vi "ParseAllClasses.vi"(8 "error in (no error)":errorcluster, 10 "baseClass":refnum<class "baseClass.lvclass">, 11 "CS in":refnum<class "CS.lvclass">) -> (0 "error out":errorcluster, 2 "AllClasses":refnum<class "baseClass.lvclass">[](array[class]), 3 "CS out":refnum<class "CS.lvclass">)   [LabVIEW 2013, in "CS.lvclass"]
uses:
  CS.lvclass
  baseClass/baseClass.lvclass
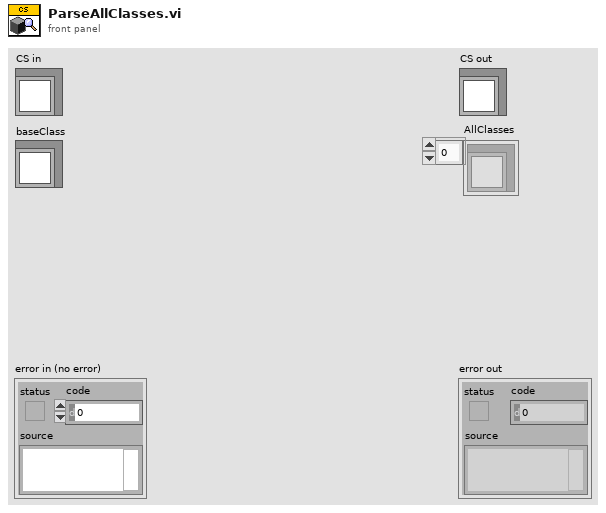
[diagram p1: front panel]
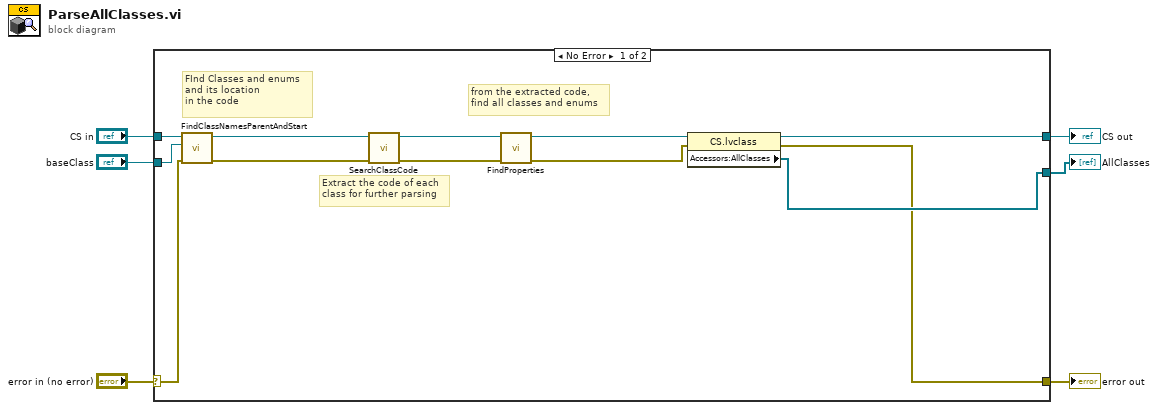
[diagram p0: block diagram]
diagram:
  n1 = case shown="No Error" "error in (no error)" {
    selector: "error in (no error)" -> [w12 w20]
    tunnel: [w11 w20] -> w6
    tunnel: [w15 _] -> w5
    tunnel: [w16 w19] -> w4
    tunnel: "baseClass" -> [w17 _]
    tunnel: "CS in" -> [w18 w19]
    frame No Error {
      # "from the extracted code,\nfind all classes and enums"
      # "Extract the code of each\nclass for further parsing"
      # "FInd Classes and enums\nand its location \nin the code"
      n2 = call "FindClassNamesParentAndStart.vi"("error in (no error)"=w12, "baseClass"=w17, "CS in"=w18) -> ("error out"=w13:errorcluster, "CS out"=w14:refnum<class "CS.lvclass">)  [unwired: 7 in]
      n3 = call-dynamic "SearchClassCode.vi"("error in (no error)"=w13, "CS in"=w14) -> ("error out"=w7:errorcluster, "CS out"=w10:refnum<class "CS.lvclass">)  [unwired: 8 in]
      n4 = call-dynamic "FindProperties.vi"("error in (no error)"=w7, "CS in"=w10) -> ("error out"=w8:errorcluster, "CS out"=w9:refnum<class "CS.lvclass">)  [unwired: 8 in]
      n5 = property class="CS.lvclass"(reference=w9, error in=w8) -> (reference out=w16:refnum<class "CS.lvclass">, error out=w11:errorcluster, "Accessors:AllClasses"=w15:refnum<class "baseClass.lvclass">[])
    }
    frame Error {
    }
  }
  "error out" <- w6
  "CS out" <- w4
  "AllClasses" <- w5
